vi "6. ProjectorScreen_StateMachine.vi"() -> ()   [LabVIEW 2019]
panel:
  in  "Stop Button":bool
  out "state":enum16{"Stop", "up", "down", "Top", "Bottom"}(ring)
  in  "Down Button":bool
  in  "Up Button":bool
  out "pos":i8(slide)
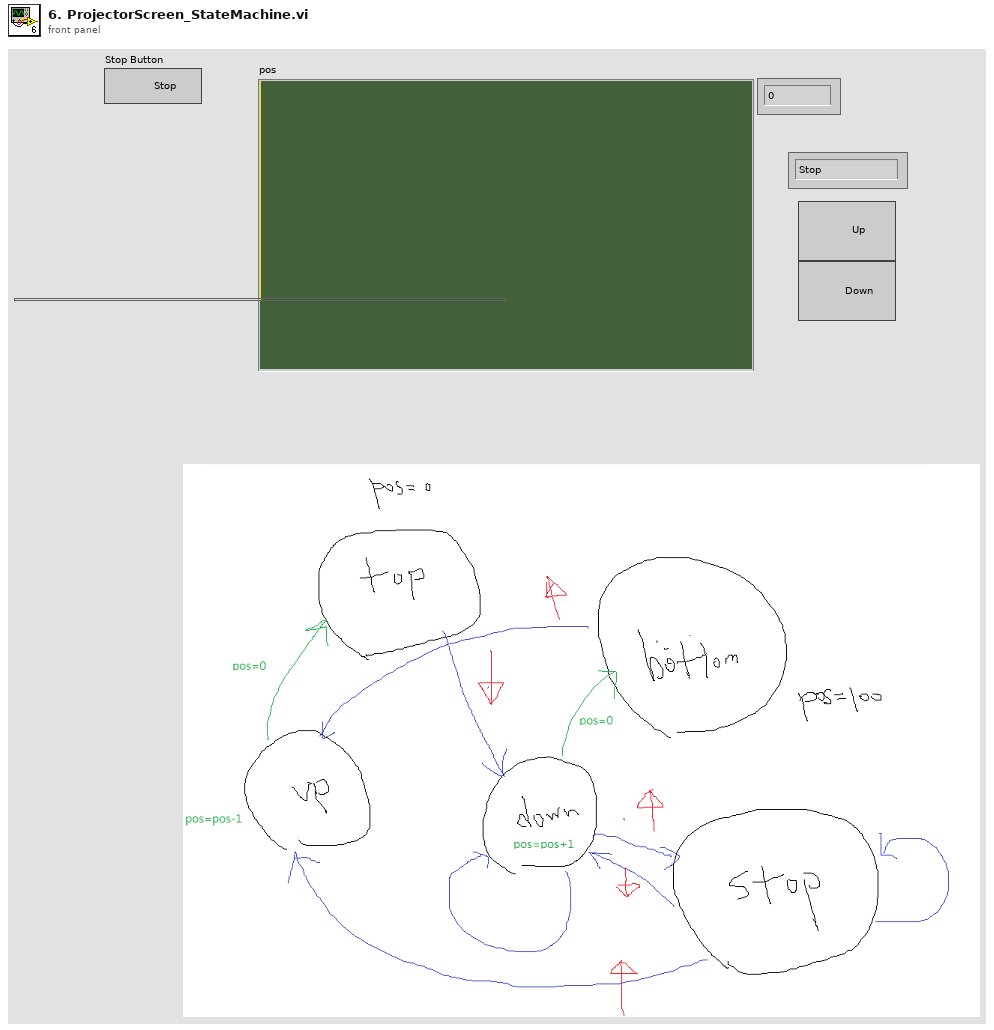
[diagram p1: front panel]
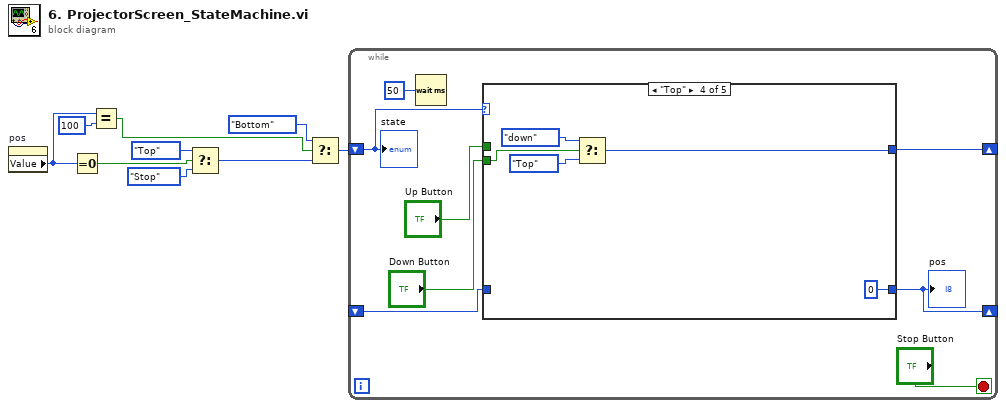
[diagram p0: block diagram]
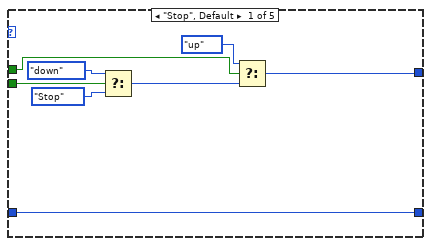
[diagram p2: hidden frame]
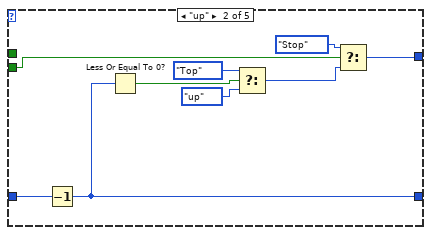
[diagram p3: hidden frame]
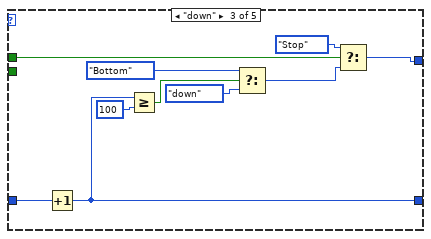
[diagram p4: hidden frame]
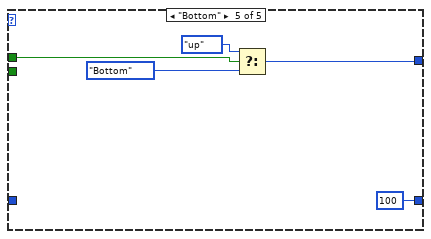
[diagram p5: hidden frame]
diagram:
  n1 = property on="pos" class="Slide (strict)"() -> ("Value"=w9:i8)  [unwired: 2 in, 2 out]
  n2 = Equal To 0?(x=w9) -> (x = 0?=w7:bool)
  n3 = Equal?(x=w9, y=i8 100) -> (x = y?=w5:bool)
  n4 = Select(t=enum16{"Stop", "up", "down", "Top", "Bottom"}."Top", s=w7, f=enum16{"Stop", "up", "down", "Top", "Bottom"}."Stop") -> (s? t:f=w3:enum16{"Stop", "up", "down", "Top", "Bottom"})
  n5 = Select(t=enum16{"Stop", "up", "down", "Top", "Bottom"}."Bottom", s=w5, f=w3) -> (s? t:f=w1:enum16{"Stop", "up", "down", "Top", "Bottom"})
  n6 = while {
    shift-right: [w16] -> _
    shift-left: w1 -> [w17]
    shift-right: [w10] -> _
    shift-left: _ -> [w11]
    stop <- "Stop Button" stop-if-true
    n7 = Wait (ms)(milliseconds to wait=u32 50) -> ()  [unwired: 1 out]
    n8 = case shown="\"Top\"" w17 {
      tunnel: [w18 w26 w36 i8 0 ("pos") i8 100 ("pos")] -> w10
      tunnel: [w23 w27 w41 w47 w51] -> w16
      tunnel: "Down Button" -> [w21 w28 _ w46 _]
      tunnel: w11 -> [w18 w29 w44 _ _]
      tunnel: "Up Button" -> [w24 _ w43 _ w53]
      frame "Stop", Default {
        n9 = Select(t=enum16{"Stop", "up", "down", "Top", "Bottom"}."down", s=w21, f=enum16{"Stop", "up", "down", "Top", "Bottom"}."Stop") -> (s? t:f=w20:enum16{"Stop", "up", "down", "Top", "Bottom"})
        n10 = Select(t=enum16{"Stop", "up", "down", "Top", "Bottom"}."up", s=w24, f=w20) -> (s? t:f=w23:enum16{"Stop", "up", "down", "Top", "Bottom"})
      }
      frame "up" {
        n11 = Decrement(x=w29) -> (x-1=w26:i8)
        n12 = Less Or Equal To 0?(x=w26) -> (x <= 0?=w33:bool)
        n13 = Select(t=enum16{"Stop", "up", "down", "Top", "Bottom"}."Top", s=w33, f=enum16{"Stop", "up", "down", "Top", "Bottom"}."up") -> (s? t:f=w30:enum16{"Stop", "up", "down", "Top", "Bottom"})
        n14 = Select(t=enum16{"Stop", "up", "down", "Top", "Bottom"}."Stop", s=w28, f=w30) -> (s? t:f=w27:enum16{"Stop", "up", "down", "Top", "Bottom"})
      }
      frame "down" {
        n15 = Increment(x=w44) -> (x+1=w36:i8)
        n16 = Greater Or Equal?(x=w36, y=i8 100 ("x")) -> (x >= y?=w37:bool)
        n17 = Select(t=enum16{"Stop", "up", "down", "Top", "Bottom"}."Bottom", s=w37, f=enum16{"Stop", "up", "down", "Top", "Bottom"}."down") -> (s? t:f=w38:enum16{"Stop", "up", "down", "Top", "Bottom"})
        n18 = Select(t=enum16{"Stop", "up", "down", "Top", "Bottom"}."Stop", s=w43, f=w38) -> (s? t:f=w41:enum16{"Stop", "up", "down", "Top", "Bottom"})
      }
      frame "Top" {
        n19 = Select(t=enum16{"Stop", "up", "down", "Top", "Bottom"}."down", s=w46, f=enum16{"Stop", "up", "down", "Top", "Bottom"}."Top") -> (s? t:f=w47:enum16{"Stop", "up", "down", "Top", "Bottom"})
      }
      frame "Bottom" {
        n20 = Select(t=enum16{"Stop", "up", "down", "Top", "Bottom"}."up", s=w53, f=enum16{"Stop", "up", "down", "Top", "Bottom"}."Bottom") -> (s? t:f=w51:enum16{"Stop", "up", "down", "Top", "Bottom"})
      }
    }
    "pos" <- w10
    "state" <- w17
  }
